vi "Add Terminals.vi"(8 "error in":errorcluster, 9 "terminal names":string[](array[string]), 10 "terminal addresses":T2[](array[typedef]), 11 "port in":T1 format="%.0x") -> (0 "error out":errorcluster, 3 "port out":T1 format="%.0x")   [LabVIEW 2020, in "Ballard MIL-STD-1553 Scripting.lvlib"]
uses:
  Ballard MIL-STD-1553 Scripting.lvlib
  Shared/Address.ctl
  <vilib>/NI VeriStand/Custom Device API/Custom Device Item Ref.ctl
  <vilib>/NI VeriStand/Custom Device API/Custom Device API.lvlib
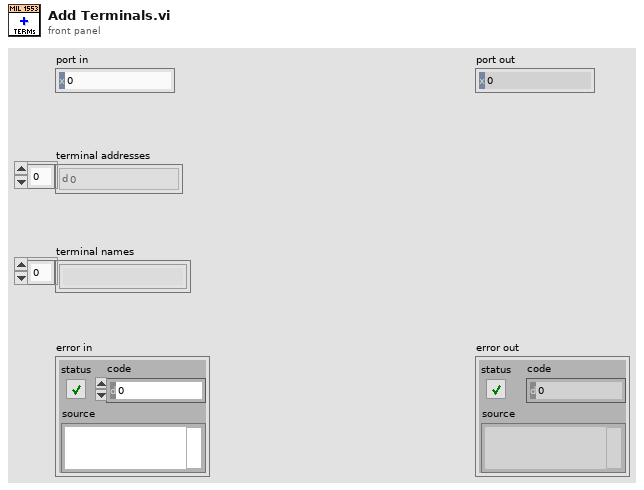
[diagram p1: front panel]
types:
  T1 = typedef "Custom Device API.lvlib/Custom Device Item Ref.ctl" = u64
  T2 = typedef "Address.ctl" = u16
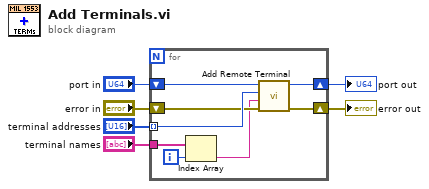
[diagram p0: block diagram]
diagram:
  n1 = for {
    shift-right: [w11] -> w3
    shift-left: "error in" -> [w12]
    tunnel: "terminal addresses" -> [w14] mode=indexing
    shift-right: [w10] -> w4
    shift-left: "port in" -> [w13]
    tunnel: "terminal names" -> [w8]
    i -> [w7]
    n2 = Index Array(array=w8, index=w7) -> (element=w9:string)
    n3 = call "Add Remote Terminal.vi"("error in"=w12, "terminal name"=w9, "terminal address"=w14, "port in"=w13) -> ("error out"=w11:errorcluster, "port out"=w10:T1)  [unwired: 5 in, 1 out]
  }
  "port out" <- w4
  "error out" <- w3
